vi "Replay Data from History.vi"(8 "error in (no error)":errorcluster, 10 "Data in":string[](array[string]), 11 "Data in":T1={"Class"={"Ants"=refnum, "Layer"=refnum, "Templates"=refnum, "Icon"=refnum, "Glyph"=refnum, "Settings"=refnum, "Tools"=refnum}, "Ref"={"Add Layer"=refnum, "Remove Layer"=refnum, "Line Text"=[], "Body Text Spec"=refnum, "DNL_Font"=refnum, "glyph path str"=refnum, "templates path str"=refnum, "Arrow Up"=refnum, "Arrow Down"=refnum, "IE VI Ref"=refnum, "Glyphs tree"=refnum, "Templates tree"=refnum, "Layer Icon Text"=refnum, "Layer Template"=refnum, "Clipboard"=refnum, "BW icon in"=refnum, "Color icon in"=refnum, "Layer Clust"=refnum, "Body Text"=refnum, "DNL_Framework Templates"=refnum, "Search Templates"=refnum, "TextMarker"=refnum, "Tab Control"=refnum, "Search Glyphs"=refnum, "Line Color"=refnum, "DNL_Glyphs []"=refnum, "Fill Color"=refnum, "Tools"=refnum, "Glyphs tree"=refnum, "Icon"=refnum, "Preview"=refnum, "Ants"=refnum, "Terminals"=refnum, "menu reference"=refnum, "LayerNames"=[], "GlyphLoadAnimation"=refnum, "TemplateLoadAnimation"=refnum, "refreshGlyphs"=refnum, "refreshTemplates"=refnum}, "Support"={"AntsRect"={"left"=0, "top"=0, "right"=0, "bottom"=0}, "Mouse Move Coords"={"Horizontal"=0, "Vertical"=0}, "Mouse Down Coords"={"Horizontal"=0, "Vertical"=0}, "Temp Coord"={"Horizontal"=0, "Vertical"=0}, "Action"=enum."Default", "Edge Color"=4914962, "Fill Color"=16860, "Mouse Down?"=FALSE, "Draft Mode?"=FALSE, "Temp Icon"=bytes[3102], "CTRL Pressed"=FALSE, "Move Selection?"=FALSE, "AntsRect Orig"={"left"=0, "top"=0, "right"=0, "bottom"=0}, "Text"="", "TM Set?"=FALSE, "Mouse inside icon?"=FALSE, "Tool (old value)"=0, "Pencil Move Color"=0, "Swap Colors?"=FALSE, "Shift pressed?"=FALSE}}) -> (0 "error out":errorcluster, 3 "Data out":T1={"Class"={"Ants"=refnum, "Layer"=refnum, "Templates"=refnum, "Icon"=refnum, "Glyph"=refnum, "Settings"=refnum, "Tools"=refnum}, "Ref"={"Add Layer"=refnum, "Remove Layer"=refnum, "Line Text"=[], "Body Text Spec"=refnum, "DNL_Font"=refnum, "glyph path str"=refnum, "templates path str"=refnum, "Arrow Up"=refnum, "Arrow Down"=refnum, "IE VI Ref"=refnum, "Glyphs tree"=refnum, "Templates tree"=refnum, "Layer Icon Text"=refnum, "Layer Template"=refnum, "Clipboard"=refnum, "BW icon in"=refnum, "Color icon in"=refnum, "Layer Clust"=refnum, "Body Text"=refnum, "DNL_Framework Templates"=refnum, "Search Templates"=refnum, "TextMarker"=refnum, "Tab Control"=refnum, "Search Glyphs"=refnum, "Line Color"=refnum, "DNL_Glyphs []"=refnum, "Fill Color"=refnum, "Tools"=refnum, "Glyphs tree"=refnum, "Icon"=refnum, "Preview"=refnum, "Ants"=refnum, "Terminals"=refnum, "menu reference"=refnum, "LayerNames"=[], "GlyphLoadAnimation"=refnum, "TemplateLoadAnimation"=refnum, "refreshGlyphs"=refnum, "refreshTemplates"=refnum}, "Support"={"AntsRect"={"left"=0, "top"=0, "right"=0, "bottom"=0}, "Mouse Move Coords"={"Horizontal"=0, "Vertical"=0}, "Mouse Down Coords"={"Horizontal"=0, "Vertical"=0}, "Temp Coord"={"Horizontal"=0, "Vertical"=0}, "Action"=enum."Default", "Edge Color"=4914962, "Fill Color"=16860, "Mouse Down?"=FALSE, "Draft Mode?"=FALSE, "Temp Icon"=bytes[3102], "CTRL Pressed"=FALSE, "Move Selection?"=FALSE, "AntsRect Orig"={"left"=0, "top"=0, "right"=0, "bottom"=0}, "Text"="", "TM Set?"=FALSE, "Mouse inside icon?"=FALSE, "Tool (old value)"=0, "Pencil Move Color"=0, "Swap Colors?"=FALSE, "Shift pressed?"=FALSE}})   [LabVIEW 2021]
uses:
  <vilib>/LabVIEW Icon API/lv_icon/Controls/Graphic.ctl
  <vilib>/LabVIEW Icon API/lv_icon/Controls/BodyText.ctl
  <vilib>/LabVIEW Icon API/lv_icon/Controls/Font.ctl
  <vilib>/LabVIEW Icon API/lv_icon/Controls/Alignment.ctl
  <resource>/plugins/NIIconEditor/Controls/IE Data.ctl
  <resource>/plugins/NIIconEditor/Class/Ants/Ants.lvclass
  <resource>/plugins/NIIconEditor/Class/FakedArray/FakedArray.lvclass
  <resource>/plugins/NIIconEditor/Class/Icon Library/Glyph.lvclass
  <resource>/plugins/NIIconEditor/Class/Settings/Settings.lvclass
  <resource>/plugins/NIIconEditor/Class/Tools/Tools Paint.lvclass
  <vilib>/LabVIEW Icon API/lv_icon/Classes/Icon/Icon.lvclass
  <resource>/plugins/NIIconEditor/Controls/IE Classes.ctl
  <resource>/plugins/NIIconEditor/Controls/References Cluster.ctl
  <resource>/plugins/NIIconEditor/Controls/SupportClass.ctl
  <vilib>/Utility/miscctls.llb/LVPoint32TypeDef.ctl
  <resource>/plugins/NIIconEditor/Controls/SupportClass_Action.ctl
  <vilib>/LabVIEW Icon API/lv_icon/Controls/IEColor.ctl
  <vilib>/LabVIEW Icon API/lv_icon/Controls/Layer.ctl
panel:
  in  "Body Text 2":T8={"Line 1 text"="", "Line 2 text"="", "Line 3 text"="", "Line 4 text"="", "Line 1 color"=0, "Line 2 color"=0, "Line 3 color"=0, "Line 4 color"=0, "Body Text Spec"={"Font"="", "Alignment"=0, "Size"=3}, "Center text vertically"=FALSE, "Capitalize Text"=FALSE} {"Body Text Spec"."Alignment" items=["left", "center", "right"]}
  in  "?":T11
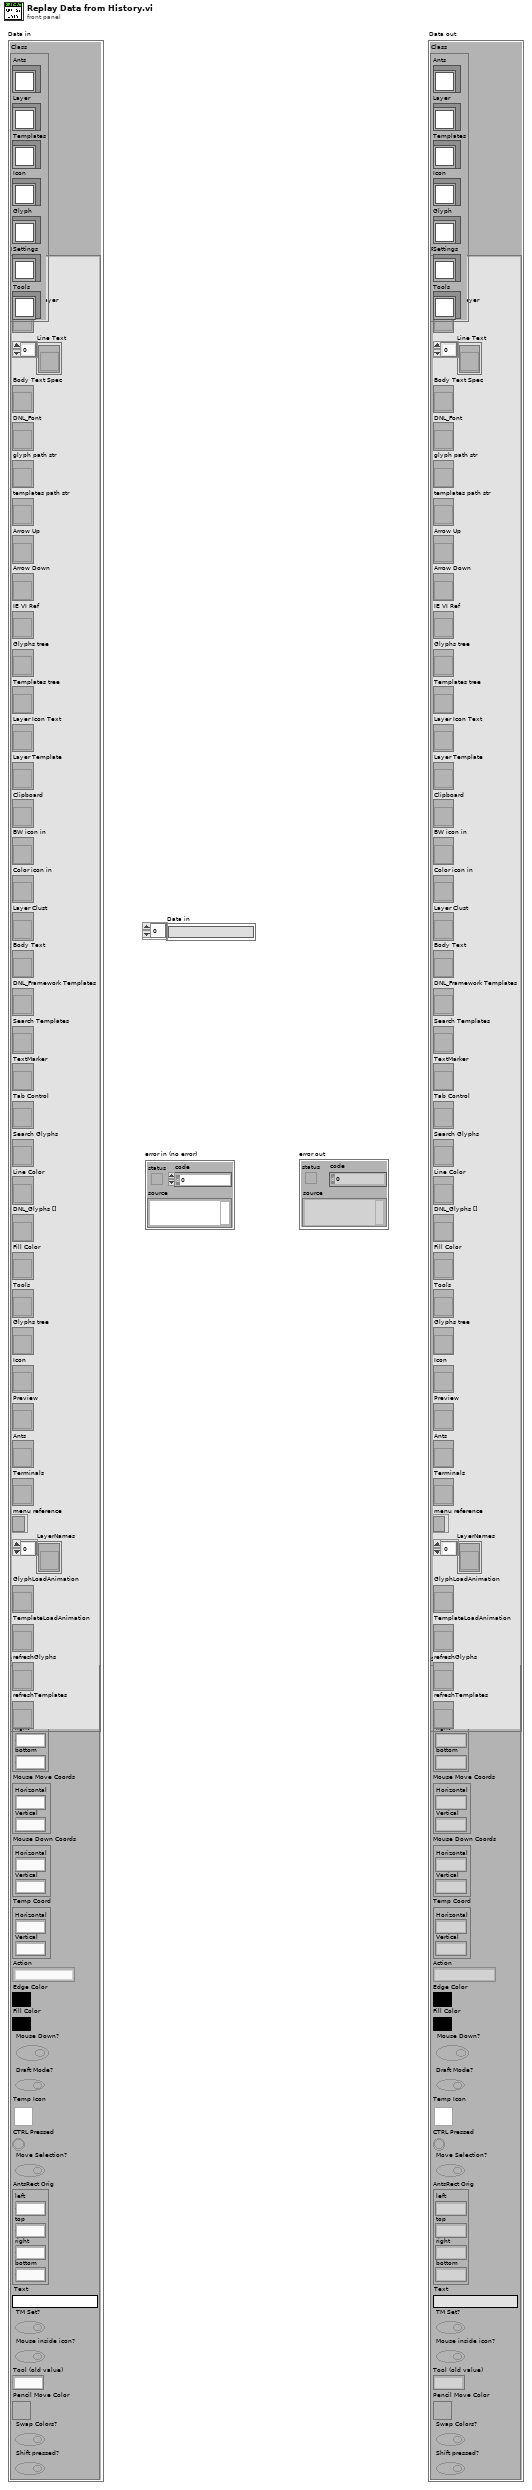
[diagram p1: front panel]
types:
  T1 = typedef "IE Data.ctl" = cluster{"Class":T2, "Ref":T3, "Support":T4}
  T2 = typedef "IE Classes.ctl" = cluster{"Ants":refnum<class "Ants.lvclass">, "Layer":refnum<class "FakedArray.lvclass">, "Templates":refnum<class "FakedArray.lvclass">, "Icon":refnum<class "Icon.lvclass">, "Glyph":refnum<class "Glyph.lvclass">, "Settings":refnum<class "Settings.lvclass">, "Tools":refnum<class "Tools Paint.lvclass">}
  T3 = typedef "References Cluster.ctl" = cluster{"Add Layer":refnum<vi>, "Remove Layer":refnum<vi>, "Line Text":refnum<vi>[], "Body Text Spec":refnum<vi>, "DNL_Font":refnum<vi>, "glyph path str":refnum<vi>, "templates path str":refnum<vi>, "Arrow Up":refnum<vi>, "Arrow Down":refnum<vi>, "IE VI Ref":refnum<vi>, "Glyphs tree":refnum<vi>, "Templates tree":refnum<vi>, "Layer Icon Text":refnum<vi>, "Layer Template":refnum<vi>, "Clipboard":refnum<vi>, "BW icon in":refnum<vi>, "Color icon in":refnum<vi>, "Layer Clust":refnum<vi>, "Body Text":refnum<vi>, "DNL_Framework Templates":refnum<vi>, "Search Templates":refnum<vi>, "TextMarker":refnum<vi>, "Tab Control":refnum<vi>, "Search Glyphs":refnum<vi>, "Line Color":refnum<vi>, "DNL_Glyphs []":refnum<vi>, "Fill Color":refnum<vi>, "Tools":refnum<vi>, "Glyphs tree":refnum<vi>, "Icon":refnum<vi>, "Preview":refnum<vi>, "Ants":refnum<vi>, "Terminals":refnum<vi>, "menu reference":refnum<k9>, "LayerNames":refnum<vi>[], "GlyphLoadAnimation":refnum<vi>, "TemplateLoadAnimation":refnum<vi>, "refreshGlyphs":refnum<vi>, "refreshTemplates":refnum<vi>}
  T4 = typedef "SupportClass.ctl" = cluster{"AntsRect":cluster{"left":i16, "top":i16, "right":i16, "bottom":i16}, "Mouse Move Coords":T5, "Mouse Down Coords":T5, "Temp Coord":T5, "Action":T6, "Edge Color":T7, "Fill Color":T7, "Mouse Down?":bool, "Draft Mode?":bool, "Temp Icon":picture, "CTRL Pressed":bool, "Move Selection?":bool, "AntsRect Orig":cluster{"left":i16, "top":i16, "right":i16, "bottom":i16}, "Text":string, "TM Set?":bool, "Mouse inside icon?":bool, "Tool (old value)":u32, "Pencil Move Color":u32, "Swap Colors?":bool, "Shift pressed?":bool}
  T5 = typedef "LVPoint32TypeDef.ctl" = cluster{"Horizontal":i32, "Vertical":i32}
  T6 = typedef "SupportClass_Action.ctl" = enum16{"Default", "Move Selection", "Glyph Library", "Tool"}
  T7 = typedef "IEColor.ctl" = u32
  T8 = typedef "BodyText.ctl" = cluster{"Line 1 text":string, "Line 2 text":string, "Line 3 text":string, "Line 4 text":string, "Line 1 color":u32, "Line 2 color":u32, "Line 3 color":u32, "Line 4 color":u32, "Body Text Spec":cluster{"Font":T9, "Alignment":T10, "Size":u8}, "Center text vertically":bool, "Capitalize Text":bool}
  T9 = typedef "Font.ctl" = string
  T10 = typedef "Alignment.ctl" = u16
  T11 = typedef "Graphic.ctl" = cluster{"Rectangle":cluster{"left":i16, "top":i16, "right":i16, "bottom":i16}, "Path":path, "Image":picture, "Filter":string, "FileName":string}
  T12 = typedef "Layer.ctl" = cluster{"LayerIcon":picture, "LayerName":string, "Opacity":u8, "Visibility?":bool}
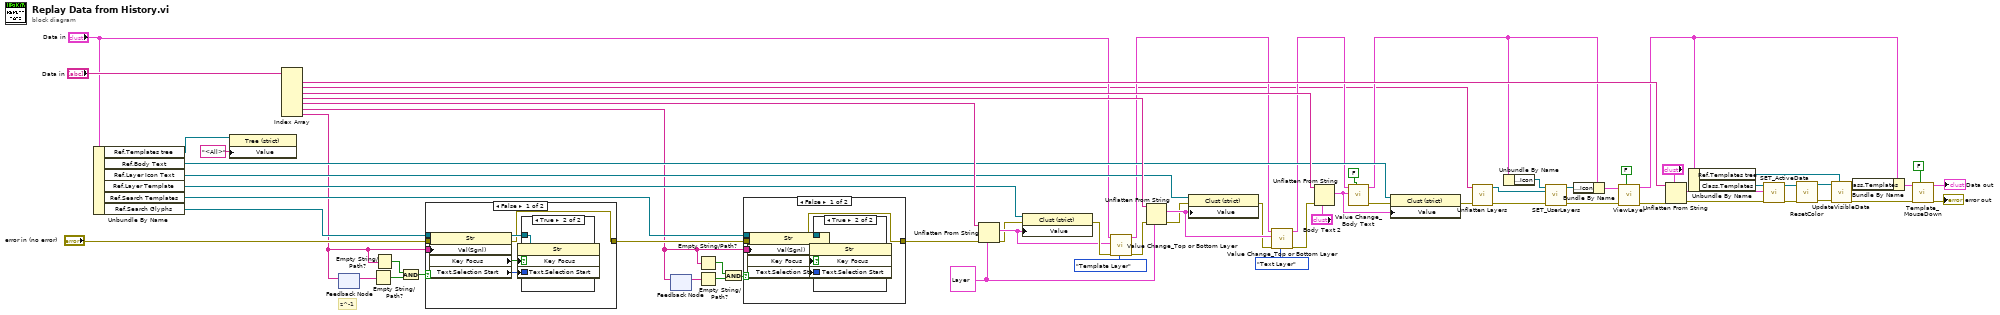
[diagram p0: block diagram]
diagram:
  w50 = T12 {"LayerIcon"=bytes[3102], "LayerName"="", "Opacity"=100, "Visibility?"=TRUE}
  # "z^-1"
  n1 = Unbundle By Name("Data in") -> ("Ref.Templates tree"=w40:refnum<vi>, "Ref.Body Text"=w52:refnum<vi>, "Ref.Layer Icon Text"=w53:refnum<vi>, "Ref.Layer Template"=w54:refnum<vi>, "Ref.Search Templates"=w13:refnum<vi>, "Ref.Search Glyphs"=w15:refnum<vi>)
  n2 = property class="Tree (strict)"(reference=w40, "Value"="<All>") -> ()  [unwired: 1 in, 2 out]
  n3 = Index Array(array="Data in") -> (element #1=w57:string, element #2=w16:string, element #3=w68:string, element #4=w69:string, element #5=w70:string, element #6=w3:string, element #7=w7:string)  [unwired: 7 in]
  n4 = feedback-in #1(w7) -> ()
  n5 = feedback #1() -> (w8:string)  [unwired: 1 in]
  n6 = Empty String/Path?(string/path=w8) -> (empty?=w10:bool)
  n7 = Empty String/Path?(string/path=w7) -> (empty?=w5:bool)
  n8 = And(x=w5, y=w10) -> (x .and. y?=w6:bool)
  n9 = case shown="False" w6 {
    tunnel: w7 -> [w77 _]
    tunnel: w15 -> [w76 _]
    tunnel: "error in (no error)" -> [w75 w81]
    tunnel: [w71 w81] -> w12
    frame False {
      n10 = property class="Str"(reference=w76, error in=w75, "Val(Sgnl)"=w77) -> (reference out=w72:refnum<vi>, error out=w71:errorcluster, "Key Focus"=w74:bool, "Text.Selection Start"=w73:u32)
      n11 = case shown="True" w74 {
        selector: w74 -> [_ w79]
        tunnel: w73 -> [_ w80]
        tunnel: w72 -> [_ w78]
        frame False {
        }
        frame True {
          n12 = property class="Str"(reference=w78, "Key Focus"=w79, "Text.Selection Start"=w80) -> ()  [unwired: 1 in, 2 out]
        }
      }
    }
    frame True {
    }
  }
  n13 = feedback #2() -> (w4:string)  [unwired: 1 in]
  n14 = feedback-in #2(w3) -> ()
  n15 = Empty String/Path?(string/path=w3) -> (empty?=w1:bool)
  n16 = Empty String/Path?(string/path=w4) -> (empty?=w9:bool)
  n17 = And(x=w1, y=w9) -> (x .and. y?=w2:bool)
  n18 = case shown="False" w2 {
    tunnel: w13 -> [w85 _]
    tunnel: w12 -> [w84 w92]
    tunnel: w3 -> [w83 _]
    tunnel: [w82 w92] -> w11
    frame False {
      n19 = property class="Str"(reference=w85, error in=w84, "Val(Sgnl)"=w83) -> (reference out=w88:refnum<vi>, error out=w82:errorcluster, "Key Focus"=w86:bool, "Text.Selection Start"=w87:u32)
      n20 = case shown="True" w86 {
        selector: w86 -> [_ w90]
        tunnel: w87 -> [_ w91]
        tunnel: w88 -> [_ w89]
        frame False {
        }
        frame True {
          n21 = property class="Str"(reference=w89, "Key Focus"=w90, "Text.Selection Start"=w91) -> ()  [unwired: 1 in, 2 out]
        }
      }
    }
    frame True {
    }
  }
  n22 = Unflatten From String(type=w50, binary string=w70, error in (no error)=w11) -> (value=w46:T12, error out=w36:errorcluster)  [unwired: 3 out]
  n23 = property class="Clust (strict)"(reference=w54, error in=w36, "Value"=w46) -> (error out=w47:errorcluster)  [unwired: 1 out]
  n24 = call <resource>:"Value Change_Top or Bottom Layer.vi"("Type"=enum16{"Template Layer", "Text Layer"}."Template Layer", "error in (no error)"=w47, "Data"=w46, "Data in"="Data in") -> ("error out"=w38:errorcluster, "Data out"=w24:T1)  [unwired: 6 out]
  n25 = Unflatten From String(type=w50, binary string=w69, error in (no error)=w38) -> (value=w44:T12, error out=w37:errorcluster)  [unwired: 3 out]
  n26 = property class="Clust (strict)"(reference=w53, error in=w37, "Value"=w44) -> (error out=w43:errorcluster)  [unwired: 1 out]
  n27 = call <resource>:"Value Change_Top or Bottom Layer.vi"("Type"=enum16{"Template Layer", "Text Layer"}."Text Layer", "error in (no error)"=w43, "Data"=w44, "Data in"=w24) -> ("error out"=w42:errorcluster, "Data out"=w21:T1)  [unwired: 6 out]
  n28 = Unflatten From String(type="Body Text 2", binary string=w68, error in (no error)=w42) -> (value=w66:T8)  [unwired: 1 in, 3 out]
  n29 = call <resource>:"Value Change_Body Text.vi"("Add to Undo?"=FALSE, "NewVal"=w66, "Data in"=w21) -> ("error out"=w64:errorcluster, "Data out"=w20:T1)  [unwired: 2 in, 5 out]
  n30 = property class="Clust (strict)"(reference=w52, error in=w64, "Value"=w66) -> (error out=w19:errorcluster)  [unwired: 1 out]
  n31 = call <resource>:"Unflatten Layers.vi"("Error In"=w19, "String"=w16) -> ("Error Out"=w18:errorcluster, "Layers"=w17:refnum<class "Layer.lvclass">[])  [unwired: 8 in]
  n32 = Unbundle By Name(w20) -> ("Class.Icon"=w35:refnum<class "Icon.lvclass">)
  n33 = call-dynamic "SET_UserLayers.vi"("error in (no error)"=w18, "Layers"=w17, "Icon.lvclass in"=w35) -> ("error out"=w27:errorcluster, "Icon.lvclass out"=w34:refnum<class "Icon.lvclass">)  [unwired: 7 in]
  n34 = Bundle By Name(cluster=w20, "Class.Icon"=w34) -> (w33:T1)
  n35 = call <resource>:"ViewLayer.vi"("Add to Undo?"=FALSE, "error in (no error)"=w27, "Data in"=w33) -> ("error out"=w51:errorcluster, "Data out"=w22:T1)  [unwired: 1 in, 6 out]
  n36 = Unflatten From String(type="?", binary string=w57, error in (no error)=w51) -> (value=w62:T11, error out=w32:errorcluster)  [unwired: 3 out]
  n37 = Unbundle By Name(w22) -> ("Ref.Templates tree"=w23:refnum<vi>, "Class.Templates"=w31:refnum<class "FakedArray.lvclass">)
  n38 = call-dynamic "SET_ActiveData.vi"("error in (no error)"=w32, "Active Data"=w62, "FakedArray.lvclass in"=w31) -> ("error out"=w59:errorcluster, "FakedArray.lvclass out"=w58:refnum<class "FakedArray.lvclass">)  [unwired: 7 out]
  n39 = call <resource>:"ResetColor.vi"("error in (no error)"=w59, "FakedArray in"=w58) -> ("error out"=w61:errorcluster, "FakedArray out"=w60:refnum<class "FakedArray.lvclass">)  [unwired: 8 out]
  n40 = call-dynamic "UpdateVisibleData.vi"("Templates tree"=w23, "error in (no error)"=w61, "FakedArray in"=w60) -> ("error out"=w26:errorcluster, "FakedArray out"=w30:refnum<class "FakedArray.lvclass">)  [unwired: 2 in, 5 out]
  n41 = Bundle By Name(cluster=w22, "Class.Templates"=w30) -> (w29:T1)
  n42 = call <resource>:"Template_MouseDown.vi"("Add to Undo?"=FALSE, "error in"=w26, "Data in"=w29) -> ("error out"=→"error out":errorcluster, "Data out"=→"Data out":T1)  [unwired: 2 in, 5 out]
